vi "SMTP Email [EXPN].vi"(8 "error in (no error)":errorcluster, 10 "address":string, 11 "smtp session":T1) -> (0 "error out":errorcluster, 1 "reply":string, 2 "reply code":i32, 3 "smtp session out":T1, 4 "recipients":string[](array[string]))   [LabVIEW 2009, in "NewNI_SMTPEmail.lvlib"]
doc: "Sends the EXPN command to the SMTP server through TCP connection described by \"connection ID\", receives reply and interprets it.\n\naddress: mailing address or list that you want expanded\n\nThis VI returns \"connection ID out,\" and the results of the error interpretation to the \"error out\" cluster."
uses:
  NewNI_SMTPEmail.lvlib
  SMTP Email Session.ctl
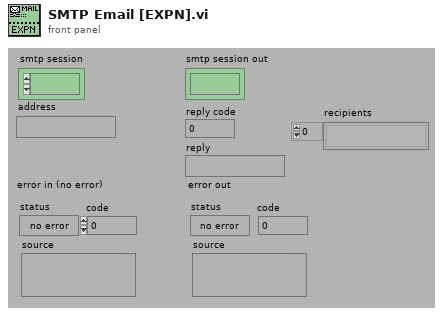
[diagram p1: front panel]
types:
  T1 = typedef "NewNI_SMTPEmail.lvlib/SMTP Email Session.ctl" = refnum<k1>
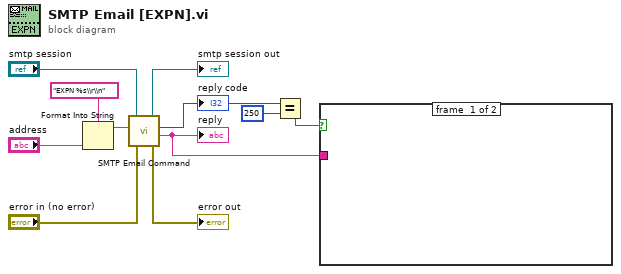
[diagram p0: block diagram]
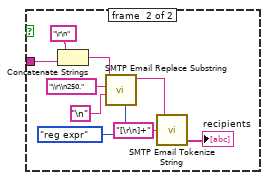
[diagram p2: hidden frame]
diagram:
  n1 = Format Into String(format string="EXPN %s\\r\\n", "address") -> (resulting string=w6:string)  [unwired: 2 in, 1 out]
  n2 = call "SMTP Email Command.vi"("error in (no error)"="error in (no error)", "command"=w6, "smtp session"="smtp session") -> ("error out"=→"error out":errorcluster, "reply"=w4:string, "reply code"=w3:i32, "smtp session out"=→"smtp session out":T1)  [unwired: 1 out]
  "reply code" <- w3
  "reply" <- w4
  n3 = Equal?(x=w3, y=250) -> (x = y?=w1:bool)
  n4 = case shown="True" w1 {
    tunnel: w4 -> [_ w15]
    frame #0 {
    }
    frame #1 {
      n5 = Concatenate Strings("\r\n", w15) -> (w18:string)
      n6 = call "SMTP Email Replace Substring.vi"("mode (literal)"=enum16{"literal", "wild card", "reg expr"}."reg expr", "replacement"="\n", "pattern"="\\r\\n250.", "text"=w18) -> ("text out"=w19:string)  [unwired: 3 in, 4 out]
      n7 = call "SMTP Email Tokenize String.vi"("delimiter ([\\s\\t\\n\\r]+)"="[\r\n]+" ("delimiter ([\\s\\t\\n\\r]+)"), "input string"=w19) -> ("token array"=→"recipients":string[])  [unwired: 3 out]
    }
  }
